vi "New format.vi"() -> ()   [LabVIEW 2015]
uses:
  Sensor configuration.ctl
  Channel type.ctl
panel:
  out "Array":path[](array[path])
  out "Names":string[](array[string])
  in  "Sensors":T1[](array[typedef])=[{"Name"="Ghz lab", "URL"="http:\\\\130.55.69.25", "Channels"=[{"type"=enum."Flow meter", "number"=6.0}]}, {"Name"="main bag", "URL"="http:\\\\130.55.69.22", "Channels"=[{"type"=enum."Flow meter", "number"=6.0}, {"type"=enum."Tank pressure", "number"=0.0}, {"type"=enum."Dewar level", "number"=1.0}]}, {"Name"="PPMS 20T", "URL"="http:\\\\130.55.69.42", "Channels"=[{"type"=enum."Flow meter", "number"=6.0}]}]
  in  "File Path Control":path=path "Z:/Data/nhmflmonitor/Helium/datalog.bin"
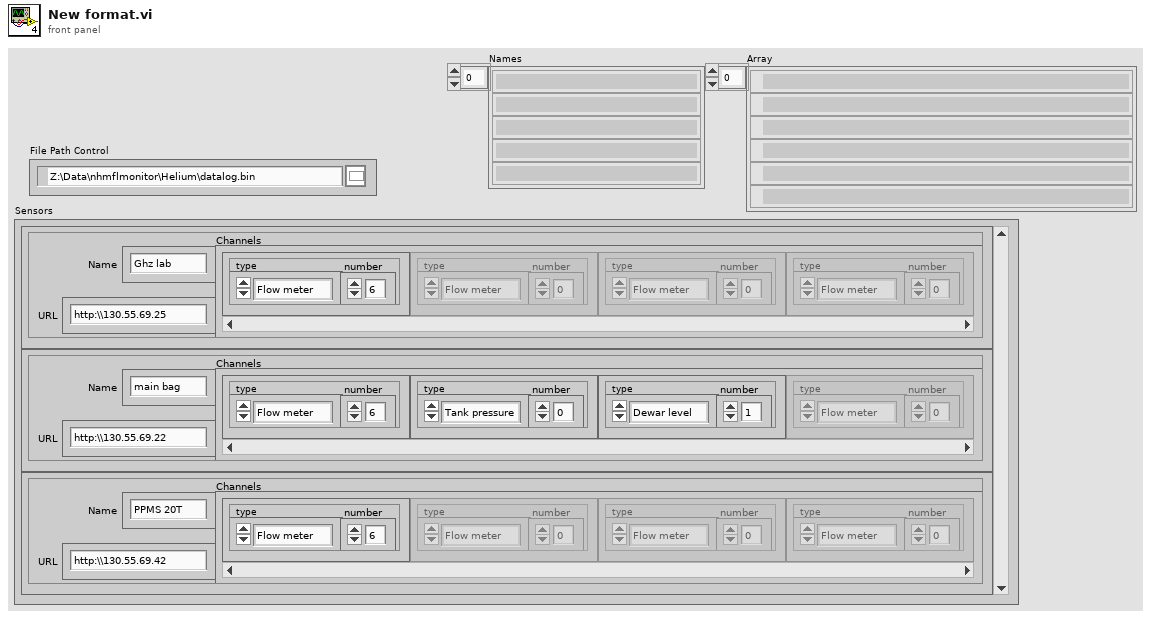
[diagram p1: front panel]
types:
  T1 = typedef "Sensor configuration.ctl" = cluster{"Name":string, "URL":string, "Channels":cluster{"type":T2, "number":dbl}[]}
  T2 = typedef "Channel type.ctl" = enum16{"Volts", "Flow meter", "Tank pressure", "Dewar level", "Raw ADC"}
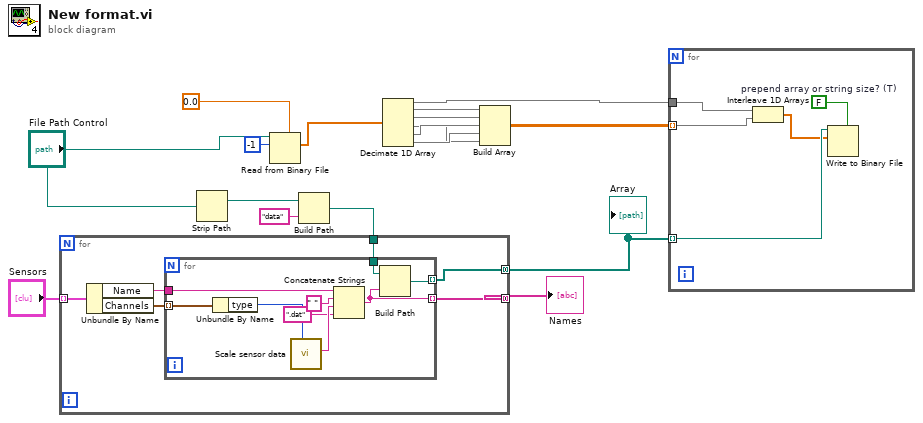
[diagram p0: block diagram]
diagram:
  n1 = Strip Path(path="File Path Control") -> (stripped path=w15:path)  [unwired: 1 out]
  n2 = Read from Binary File(5:0.0, 10:-1 ("count (1)"), 11:"File Path Control") -> (2:w9:dbl[])  [unwired: 3 in, 3 out]
  n3 = Build Path(base path=w15, name or relative path="data") -> (appended path=w13:path)
  n4 = for {
    tunnel: "Sensors" -> [w23] mode=indexing
    tunnel: [w21] -> w16 mode=concatenating
    tunnel: w13 -> [w19]
    tunnel: [w18] -> w4 mode=concatenating
    n5 = Unbundle By Name(w23) -> ("Name"=w22:string, "Channels"=w20:cluster{"type":T2, "number":dbl}[])
    n6 = for {
      tunnel: w20 -> [w30] mode=indexing
      tunnel: w22 -> [w32]
      tunnel: [w25] -> w21 mode=indexing
      tunnel: w19 -> [w26]
      tunnel: [w24] -> w18 mode=indexing
      n7 = Unbundle By Name(w30) -> ("type"=w29:T2)
      n8 = call "Scale sensor data.vi"("Channel type"=w29) -> ("Type name"=w28:string)  [unwired: 9 in, 1 out]
      n9 = Concatenate Strings(w32, " " ("string"), w28, ".dat" ("string")) -> (w25:string)
      n10 = Build Path(base path=w26, name or relative path=w25) -> (appended path=w24:path)
    }
  }
  "Names" <- w16
  "Array" <- w4
  n11 = Decimate 1D Array(w9) -> (w6:dbl[], w8:dbl[], w7:dbl[], w1:dbl[], w3:dbl[], w2:dbl[])
  n12 = Build Array(w8, w7, w3, w2, w1) -> (w5:dbl[][])
  n13 = for {
    tunnel: w6 -> [w37]
    tunnel: w5 -> [w36] mode=indexing
    tunnel: w4 -> [w35] mode=indexing
    w33 = FALSE  # prepend array or string size? (T)
    n14 = Interleave 1D Arrays(w37, w36) -> (w34:dbl[])
    n15 = Write to Binary File(file (use dialog)=w35, data=w34, 5:w33) -> ()  [unwired: 3 in, 3 out]
  }
